vi "TYPE.vi"(9 "Type":u8=35, 11 "Python in":string="import machine, utime\n\ntx = machine.Pin('Y9', machine.Pin.OUT)\nrx = machine.Pin('Y10', machine.Pin.IN)\ntx.value(b'\\x00')\nutime.sleep_ms(500)\ntx.value(1)\n\nuart = machine.UART(3)\nuart.init(baudrate=2400, bits=8, parity=None, stop=1)\n\nuart.write(0)\n") -> (3 "Python out":string="import machine, utime\n\ntx = machine.Pin('Y9', machine.Pin.OUT)\nrx = machine.Pin('Y10', machine.Pin.IN)\ntx.value(b'\\x00')\nutime.sleep_ms(500)\ntx.value(1)\n\nuart = machine.UART(3)\nuart.init(baudrate=2400, bits=8, parity=None, stop=1)\n\nuart.write(0)\nuart.write(b'\\x40\\x23\\x9C')\n")   [LabVIEW 2016]
panel:
  out "bytes added":u8[](array[numeric])=[64, 35, 156] format="%.0b"
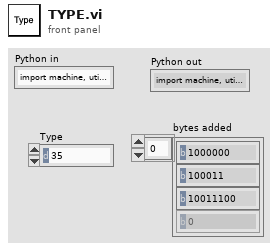
[diagram p1: front panel]
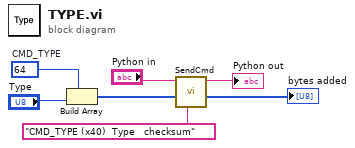
[diagram p0: block diagram]
diagram:
  w6 = u8 64  # CMD_TYPE
  n1 = Build Array(w6, "Type") -> (w3:u8[])
  n2 = call "SendCmd.vi"("Comment"="CMD_TYPE (x40)  Type   checksum", "Array In"=w3, "Python in"="Python in") -> ("Array Sent"=→"bytes added":u8[], "Python out"=→"Python out":string)  [unwired: 7 in]
